vi "Save File Extract Save Path.vi"(6 "Debug or Inv File?":T3, 7 "Extract (F)":bool, 8 "Error In":errorcluster, 9 "File Name to Save":path, 11 "File Locations In":T1) -> (0 "Error Out":errorcluster, 2 "File Locations Out":T1, 3 "Extracted File Name":path)   [LabVIEW 2019, in "Save File.lvlib"]
uses:
  Save File.lvlib
  Type Definitions/Save File Type.ctl
  File Setup (Public)/Type Definition/Save File DOE File Path Control.ctl
  File Setup (Public)/Type Definition/Save File DOE Data Save Filepaths.ctl
  File Setup.lvlib
panel:
  # "Extract File Name"
  # "Save File Name"
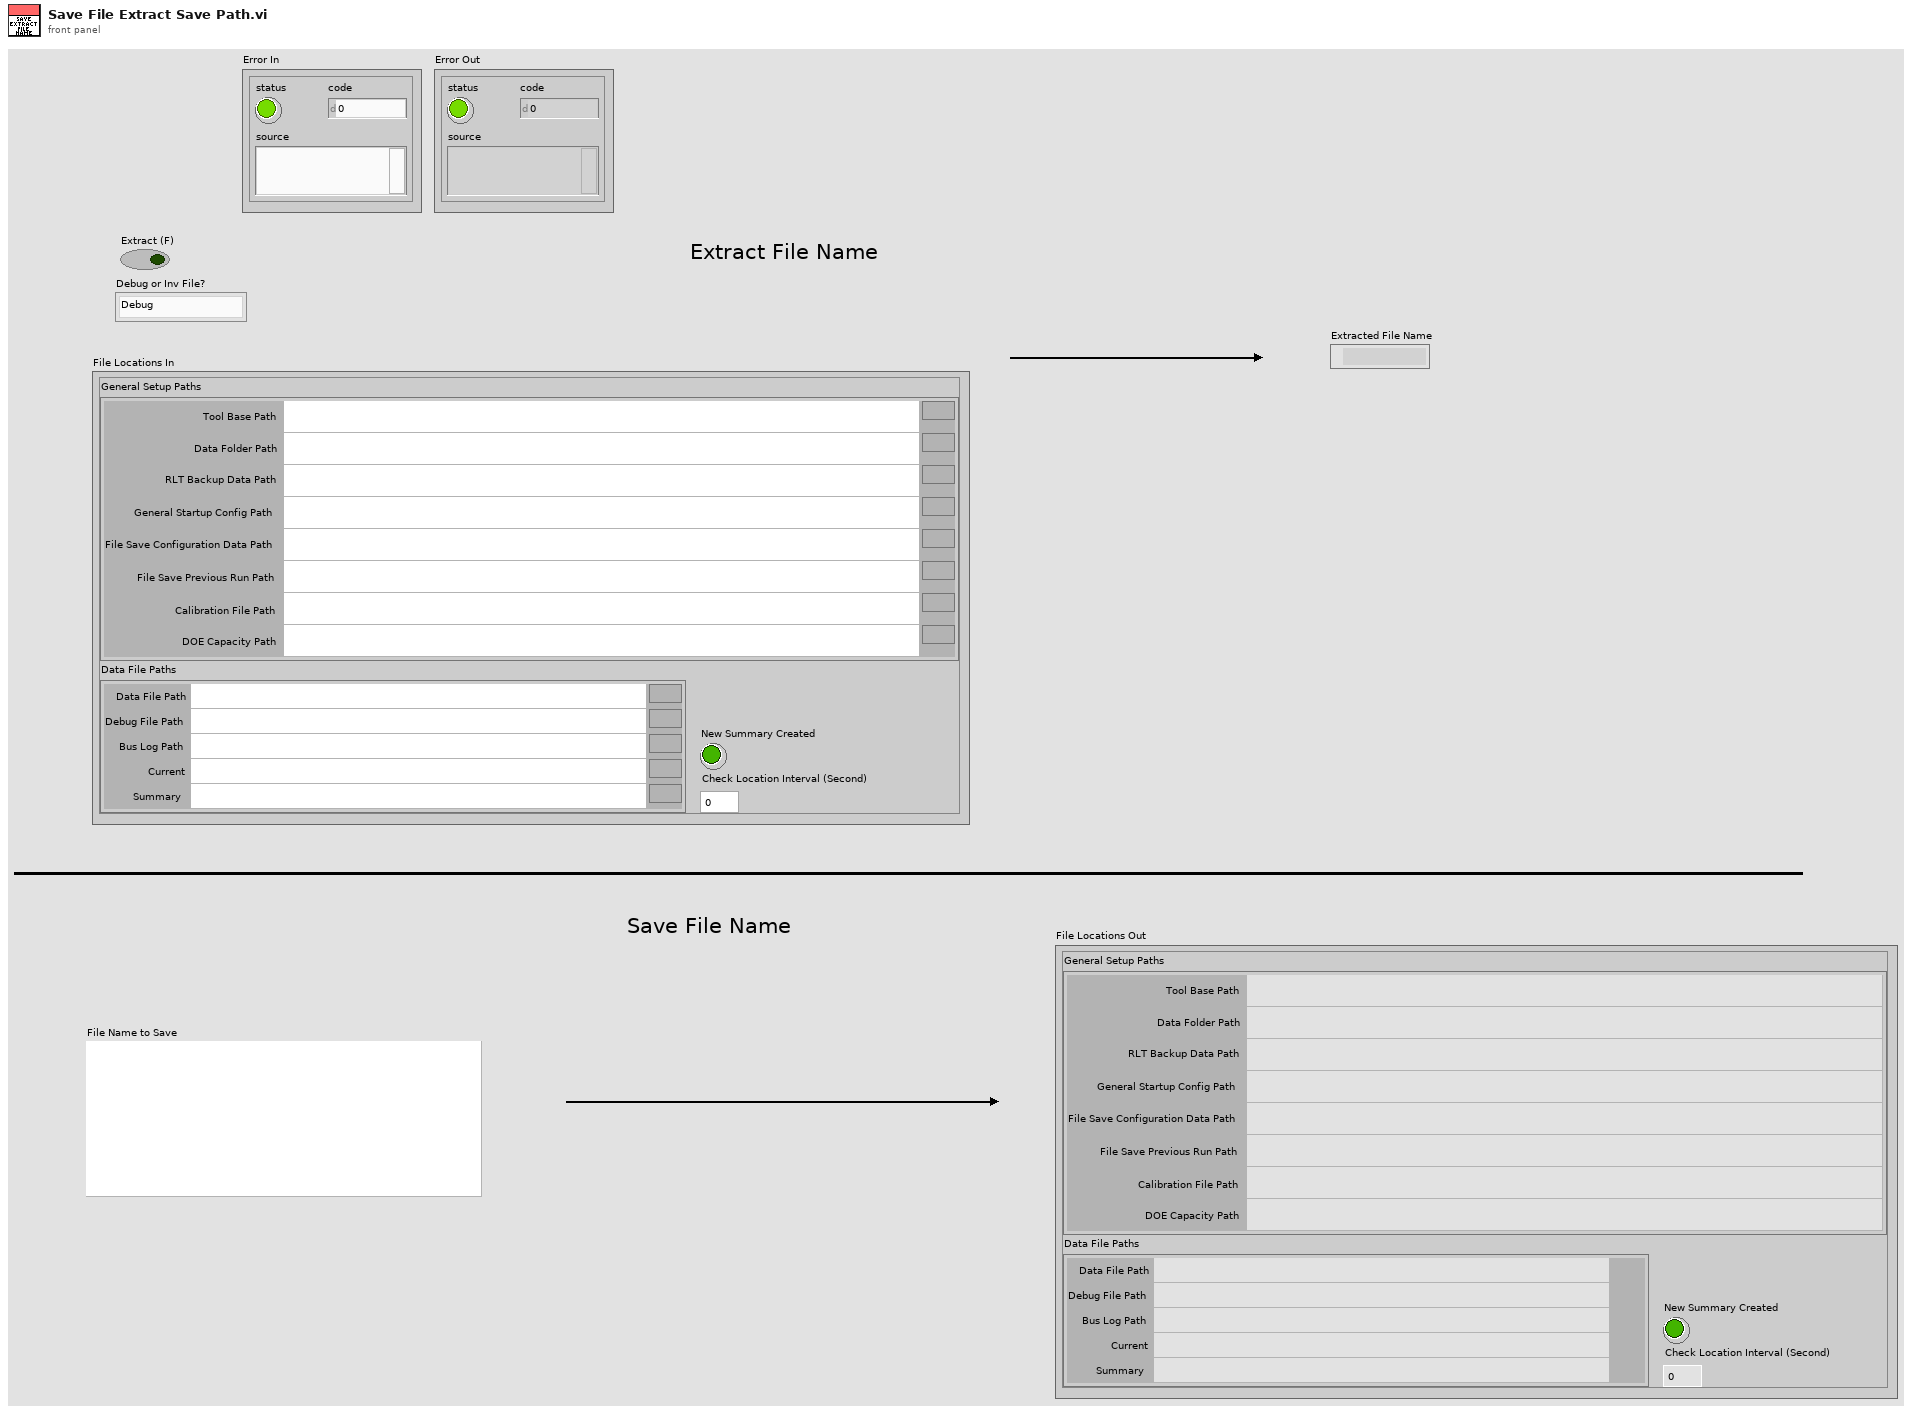
[diagram p1: front panel]
types:
  T1 = typedef "File Setup.lvlib/Save File DOE File Path Control.ctl" = cluster{"General Setup Paths":cluster{"Calibration File Path":path, "DOE Capacity Path":path, "Data Folder Path":path, "RLT Backup Data Path":path, "Tool Base Path":path, "General Startup Config Path":path, "File Save Previous Run Path":path, "File Save Configuration Data Path":path}, "Data File Paths":T2, "New Summary Created":bool, "Check Location Interval (Second)":i32}
  T2 = typedef "File Setup.lvlib/Save File DOE Data Save Filepaths.ctl" = cluster{"Data File Path":path, "Debug File Path":path, "Bus Log Path":path, "Current":path, "Summary":path}
  T3 = typedef "Save File Type.ctl" = enum16{"Debug", "Inv and MC", "Current", "Bus File"}
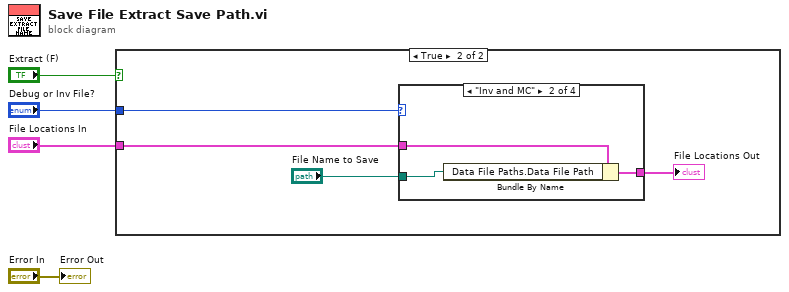
[diagram p0: block diagram]
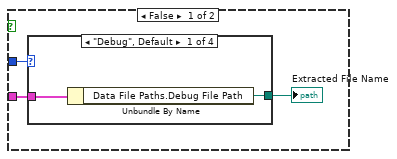
[diagram p2: hidden frame]
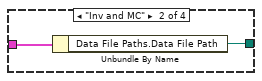
[diagram p3: hidden frame]
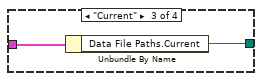
[diagram p4: hidden frame]
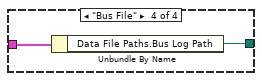
[diagram p5: hidden frame]
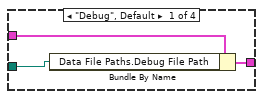
[diagram p6: hidden frame]
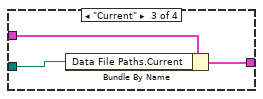
[diagram p7: hidden frame]
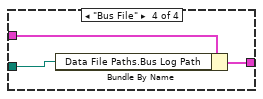
[diagram p8: hidden frame]
diagram:
  n1 = case shown="True" "Extract (F)" {
    tunnel: "File Locations In" -> [w6 w17]
    tunnel: "Debug or Inv File?" -> [w5 w18]
    frame False {
      n2 = case shown="\"Debug\", Default" w5 {
        tunnel: w6 -> [w9 w11 w12 w15]
        tunnel: [w8 w10 w13 w14] -> w7
        frame "Debug", Default {
          n3 = Unbundle By Name(w9) -> ("Data File Paths.Debug File Path"=w8:path)
        }
        frame "Inv and MC" {
          n4 = Unbundle By Name(w11) -> ("Data File Paths.Data File Path"=w10:path)
        }
        frame "Current" {
          n5 = Unbundle By Name(w12) -> ("Data File Paths.Current"=w13:path)
        }
        frame "Bus File" {
          n6 = Unbundle By Name(w15) -> ("Data File Paths.Bus Log Path"=w14:path)
        }
      }
      "Extracted File Name" <- w7
    }
    frame True {
      n7 = case shown="\"Inv and MC\"" w18 {
        tunnel: w17 -> [w22 w25 w28 w30]
        tunnel: [w21 w24 w27 w29] -> w16
        tunnel: "File Name to Save" -> [w20 w23 w26 w31]
        frame "Debug", Default {
          n8 = Bundle By Name(cluster=w22, "Data File Paths.Debug File Path"=w20) -> (w21:T1)
        }
        frame "Inv and MC" {
          n9 = Bundle By Name(cluster=w25, "Data File Paths.Data File Path"=w23) -> (w24:T1)
        }
        frame "Current" {
          n10 = Bundle By Name(cluster=w28, "Data File Paths.Current"=w26) -> (w27:T1)
        }
        frame "Bus File" {
          n11 = Bundle By Name(cluster=w30, "Data File Paths.Bus Log Path"=w31) -> (w29:T1)
        }
      }
      "File Locations Out" <- w16
    }
  }
  "Error Out" <- "Error In"
